vi "Format GUI Elements.vi"() -> ()   [LabVIEW 2018]
panel:
  in  "new element/subarray":string[](array[string])
  out "array":string[](array[string])
  out "Test Table2":string[][](table)=[["", "20"]] caption="Table"
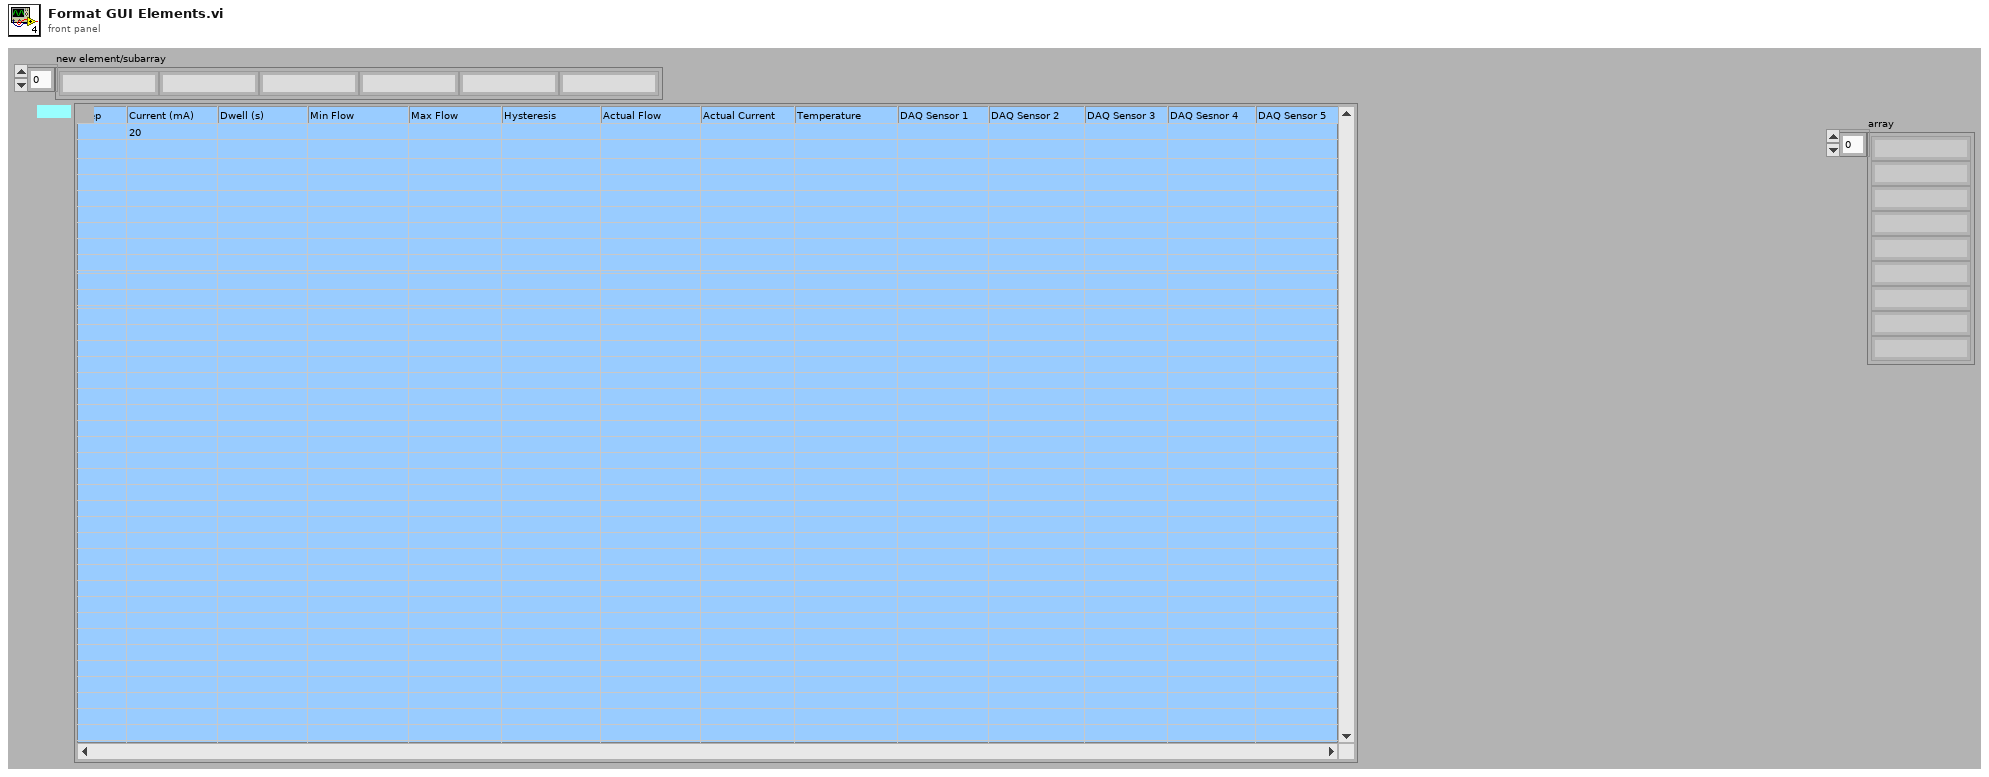
[diagram p1: front panel]
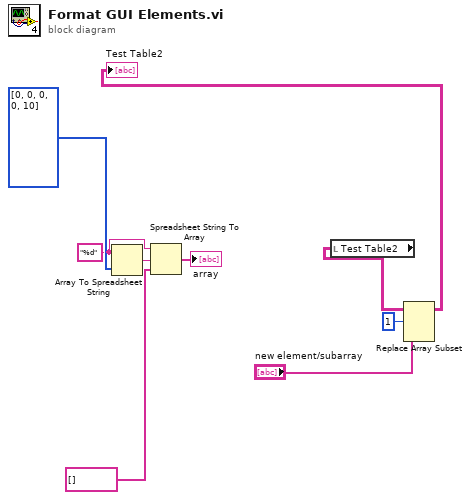
[diagram p0: block diagram]
diagram:
  w6 = "%d" ("format string")
  n1 = Array To Spreadsheet String(array=i32[] [0, 0, 0, 0, 10], 3:w6) -> (spreadsheet string=w9:string)  [unwired: 1 in]
  n2 = Spreadsheet String To Array(format string=w6, spreadsheet string=w9, array type (2D Dbl)=string[] []) -> (array=→"array":string[])  [unwired: 1 in]
  n3 = local read "Test Table2"() -> (w5:string[][])
  n4 = Replace Array Subset "Replace Array Subset"(array=w5, new element="new element/subarray", index (row)=1) -> (→"Test Table2":string[][])  [unwired: 1 in]
